vi "Configure Marker State.vi"(7 "Maker On (F)":bool, 8 "error in (no error)":errorcluster, 10 "Marker Number (1)":u32=1 min=1, 11 "SA-ESA in":refnum<class "SA-ESA.lvclass">) -> (0 "error out":errorcluster, 3 "SA-ESA out":refnum<class "SA-ESA.lvclass">)   [LabVIEW 2020, in "SA-ESA.lvclass"]
uses:
  SA-ESA.lvclass
  C:/Sandbox/Git_Sandbox/WiSpry Test Framework source code (LV20)/WiSpry Test Framework/Instruments/Instrument.lvclass
  Instrument.lvclass/Instrument.ctl
  Instrument.lvclass
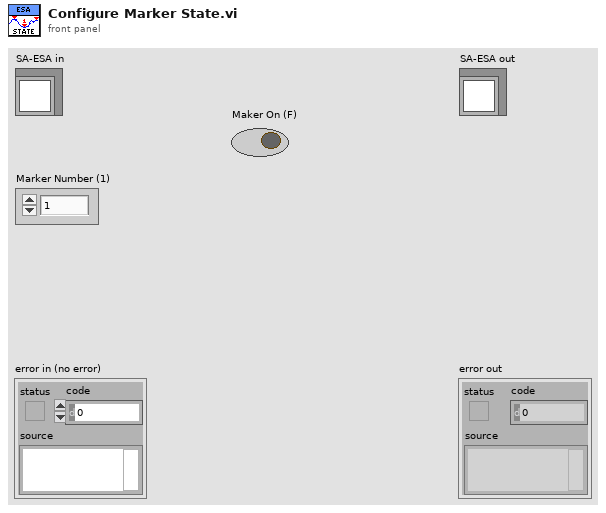
[diagram p1: front panel]
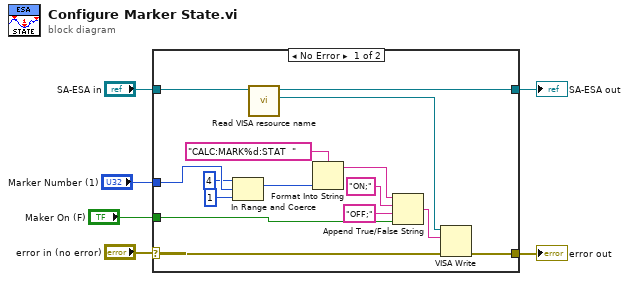
[diagram p0: block diagram]
diagram:
  n1 = case shown="No Error" "error in (no error)" {
    selector: "error in (no error)" -> [w10 w22]
    tunnel: "Marker Number (1)" -> [w20 _]
    tunnel: "SA-ESA in" -> [w21 w23]
    tunnel: "Maker On (F)" -> [w12 _]
    tunnel: [w8 w22] -> w2
    tunnel: [w7 w23] -> w1
    frame No Error {
      n2 = In Range and Coerce(upper limit=u32 4, x=w20, lower limit=u32 1) -> (coerced(x)=w17:u32)  [unwired: 1 out]
      n3 = call "Read VISA resource name.vi"("Instrument in"=w21) -> ("VISA resource name"=w11:refnum<visa-resource-name>, "Instrument out"=w7:refnum<class "SA-ESA.lvclass">)  [unwired: 9 in]
      n4 = Format Into String(format string="CALC:MARK%d:STAT  ", w17) -> (resulting string=w15:string)  [unwired: 2 in, 1 out]
      n5 = Append True/False String(1:w12, 2:"OFF;" ("false string"), 3:"ON;" ("true string"), 4:w15) -> (0:w9:string)
      n6 = VISA Write(VISA resource name=w11, write buffer=w9, error in (no error)=w10) -> (error out=w8:errorcluster)  [unwired: 2 out]
    }
    frame Error {
    }
  }
  "error out" <- w2
  "SA-ESA out" <- w1
